vi "HT3_Open.vi"(8 "error in":errorcluster, 11 "File Path":path) -> (0 "error out":errorcluster, 1 "Num Records":i64, 2 "Header":T2={"Ident"="", "Format Version"="", "Creator Name"="", "Creator Version"="", "File Time"="", "Comment"="", "Binning"=0, "Offset"=0, "AcquisitionTime (ms)"=0, "HardwareSerial"=0, "SyncDivider"=0, "Resolution (ps)"=0.0, "InpRate0"=0, "InpRate1"=0, "CFD Settings"={"Sync Level"=150, "Sync ZeroX"=10, "Sync Offset"=-1000, "Chan Settings"=[{"CHx Level"=50, "CHx ZeroX"=10, "CHx Offset"=0}, {"CHx Level"=50, "CHx ZeroX"=10, "CHx Offset"=0}, {"CHx Level"=50, "CHx ZeroX"=10, "CHx Offset"=0}, {"CHx Level"=50, "CHx ZeroX"=10, "CHx Offset"=0}]}}, 3 "refnum out":refnum<file>, 4 "Stop After (ms)":i32, 5 "Stop Reason":enum16{"timeover", "manual", "overflow"}(ring), 7 "Image Header":T1)   [LabVIEW 2010]
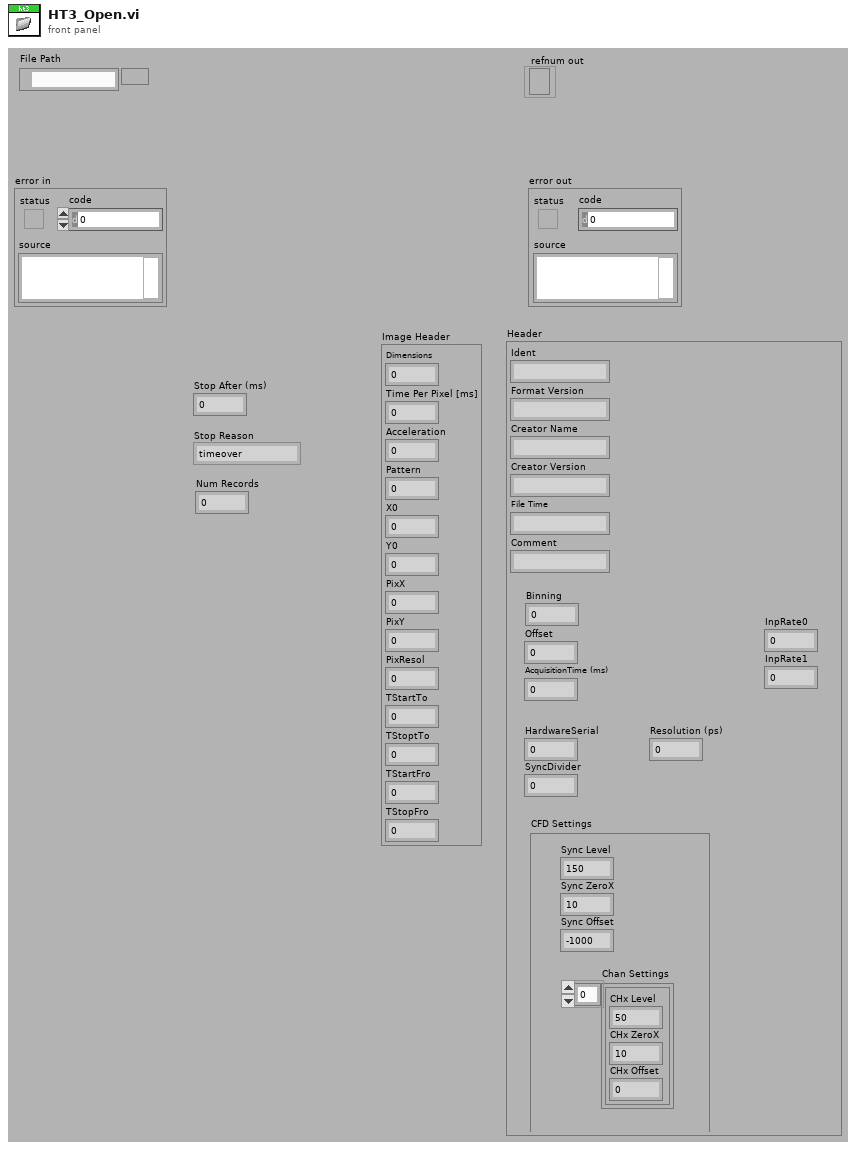
[diagram p1: front panel]
types:
  T1 = cluster{"Dimensions":i32, "Time Per Pixel [ms]":dbl, "Acceleration":i32, "Pattern":i32, "X0":sgl, "Y0":sgl, "PixX":i32, "PixY":i32, "PixResol":sgl, "TStartTo":sgl, "TStoptTo":sgl, "TStartFro":sgl, "TStopFro":sgl}
  T2 = cluster{"Ident":string, "Format Version":string, "Creator Name":string, "Creator Version":string, "File Time":string, "Comment":string, "Binning":i32, "Offset":i32, "AcquisitionTime (ms)":i32, "HardwareSerial":i32, "SyncDivider":i32, "Resolution (ps)":dbl, "InpRate0":i32, "InpRate1":i32, "CFD Settings":cluster{"Sync Level":i32, "Sync ZeroX":i32, "Sync Offset":i32, "Chan Settings":cluster{"CHx Level":i32, "CHx ZeroX":i32, "CHx Offset":i32}[]}}
  T3 = cluster{"Sync Level":i32, "Sync ZeroX":i32, "Sync Offset":i32, "Chan Settings":cluster{"CHx Level":i32, "CHx ZeroX":i32, "CHx Offset":i32}[]}
  T4 = enum16{"big-endian, network order", "native, host order", "little-endian"}
  T5 = enum16{"open", "replace", "create", "open or create", "replace or create", "replace or create with confirmation"}
  T6 = cluster{"Strings[0]":string, "Strings[1]":string, "Strings[2]":string, "Strings[3]":string, "Strings[4]":string, "Strings[5]":string}
  T7 = cluster{"[0]":i32, "[1]":i32, "[2]":i32, "[3]":i32}
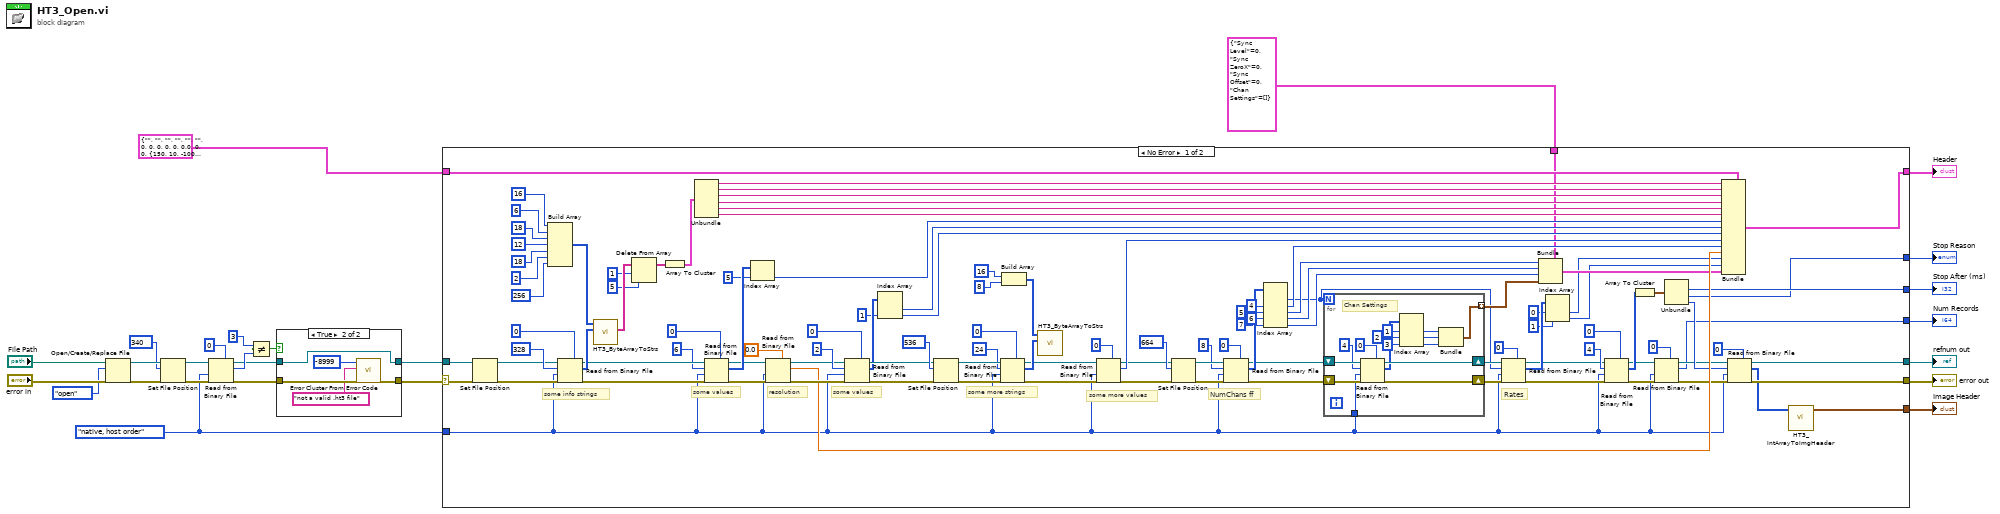
[diagram p0: block diagram]
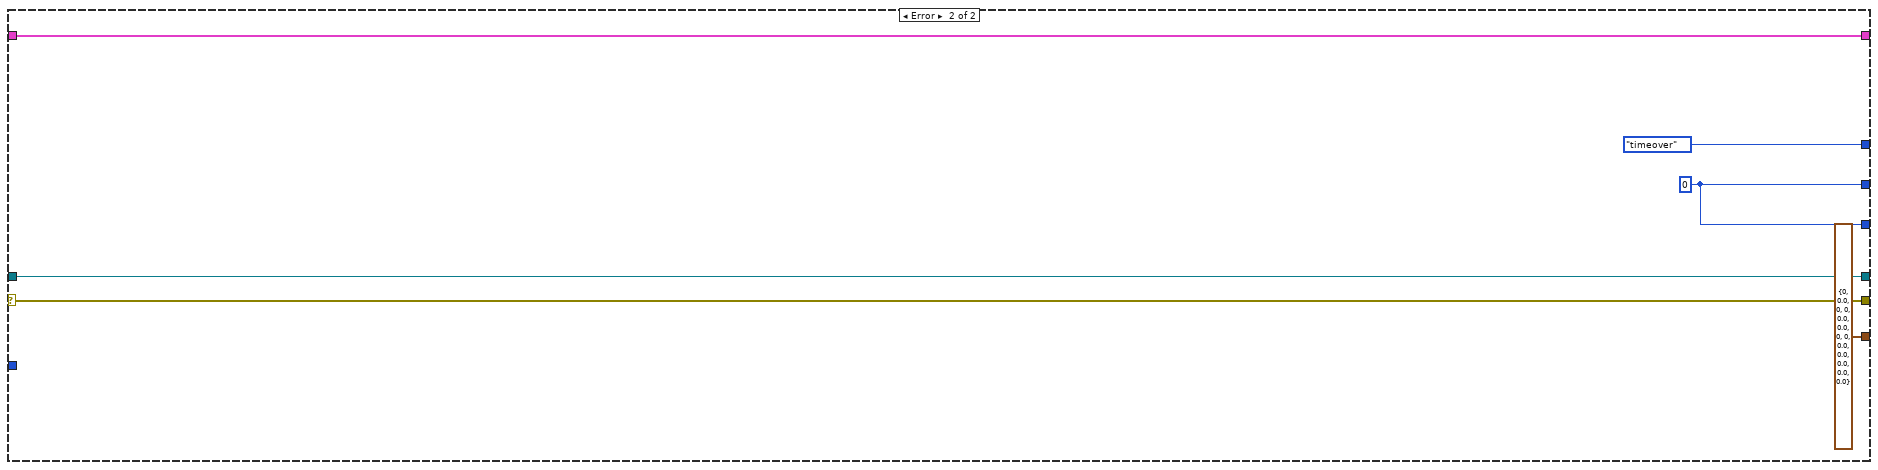
[diagram p3: hidden frame]
diagram:
  w12 = T4."native, host order" ("byte order (0:big-endian, network order)")
  n1 = Open/Create/Replace File(file path (use dialog)="File Path", error in="error in", operation (0:open)=T5."open") -> (refnum out=w15:refnum<file>, error out=w16:errorcluster)  [unwired: 4 out]
  n2 = Set File Position(offset (in bytes) (0)=i64 340, refnum=w15, error in=w16) -> (refnum out=w11:refnum<file>, error out=w13:errorcluster)  [unwired: 1 out]
  n3 = Read from Binary File(5:0, 8:w13, 9:w12, 11:w11) -> (0:w6:errorcluster, 2:w9:i32, 3:w3:refnum<file>)  [unwired: 3 out]
  n4 = Not Equal?(x=3, y=w9) -> (x != y?=w7:bool)
  n5 = case shown="True" w7 {
    tunnel: w6 -> [w28 w33]
    tunnel: [w28 w32] -> w5
    tunnel: [w27 w29] -> w4
    tunnel: w3 -> [w27 w29]
    frame False {
    }
    frame True {
      n6 = call <vilib>:"Error Cluster From Error Code.vi"("error in (no error)"=w33, "error message (\"\")"="not a valid .ht3 file" ("error message (\"\")"), "error code (0)"=-8999) -> ("error out"=w32:errorcluster)  [unwired: 1 in, 5 out]
    }
  }
  n7 = case shown="No Error" w5 {
    selector: w5 -> [w129 w167]
    tunnel: [w94 w167] -> w23
    tunnel: [w93 w166] -> w22
    tunnel: w4 -> [w127 w166]
    tunnel: w12 -> [w38 _]
    tunnel: [w120 w163] -> w21
    tunnel: [w41 enum16{"timeover", "manual", "overflow"}."timeover" ("Stop Reason")] -> w20
    tunnel: [w42 w164] -> w19
    tunnel: [w34 w164] -> w18
    tunnel: T2 {"Ident"="", "Format Version"="", "Creator Name"="", "Creator Version"="", "File Time"="", "Comment"="", "Binning"=0, "Offset"=0, "AcquisitionTime (ms)"=0, "HardwareSerial"=0, "SyncDivider"=0, "Resolution (ps)"=0.0, "InpRate0"=0, "InpRate1"=0, "CFD Settings"={"Sync Level"=150, "Sync ZeroX"=10, "Sync Offset"=-1000, "Chan Settings"=[{"CHx Level"=50, "CHx ZeroX"=10, "CHx Offset"=0}, {"CHx Level"=50, "CHx ZeroX"=10, "CHx Offset"=0}, {"CHx Level"=50, "CHx ZeroX"=10, "CHx Offset"=0}, {"CHx Level"=50, "CHx ZeroX"=10, "CHx Offset"=0}]}} ("Header") -> [w121 w163]
    tunnel: [w91 T1 {"Dimensions"=0, "Time Per Pixel [ms]"=0.0, "Acceleration"=0, "Pattern"=0, "X0"=0.0, "Y0"=0.0, "PixX"=0, "PixY"=0, "PixResol"=0.0, "TStartTo"=0.0, "TStoptTo"=0.0, "TStartFro"=0.0, "TStopFro"=0.0} ("Image Header")] -> w2
    tunnel: T3 {"Sync Level"=0, "Sync ZeroX"=0, "Sync Offset"=0, "Chan Settings"=[]} ("CFD Settings") -> [w63 _]
    frame No Error {
      # "Rates"
      # "NumChans ff"
      # "some values"
      # "resolution"
      # "some more values"
      # "some more strings"
      # "some values"
      # "some info strings"
      n8 = Set File Position(refnum=w127, error in=w129) -> (refnum out=w126:refnum<file>, error out=w128:errorcluster)  [unwired: 2 out]
      n9 = Build Array(16 ("Length"), 6 ("Length"), 18 ("Length"), 12 ("Length"), 18 ("Length"), 2 ("Length"), 256 ("Length")) -> (w136:i32[])
      n10 = Read from Binary File(5:u8 0, 8:w128, 9:w38, 10:328 ("count (1)"), 11:w126) -> (0:w131:errorcluster, 2:w144:u8[], 3:w130:refnum<file>)  [unwired: 2 out]
      n11 = call "HT3_ByteArrayToStrs.vi"("Byte Array"=w144, "Lengths"=w136) -> ("Strings"=w135:string[])  [unwired: 9 out]
      n12 = Delete From Array(array=w135, length=1, index=5) -> (array with subset deleted=w132:string[])  [unwired: 1 out]
      n13 = Array To Cluster(array=w132) -> (cluster=w119:T6)
      n14 = Unbundle(w119) -> ("Strings[0]"=w118:string, "Strings[1]"=w117:string, "Strings[2]"=w116:string, "Strings[3]"=w115:string, "Strings[4]"=w114:string, "Strings[5]"=w113:string)
      n15 = Read from Binary File(5:0, 8:w131, 9:w38, 10:6 ("count (1)"), 11:w130) -> (0:w89:errorcluster, 2:w123:i32[], 3:w88:refnum<file>)  [unwired: 2 out]
      n16 = Index Array(array=w123, index=5) -> (element=w112:i32)
      n17 = Read from Binary File(5:0.0 ("Resolution (ns)"), 8:w89, 9:w38, 11:w88) -> (0:w85:errorcluster, 2:w77:dbl, 3:w83:refnum<file>)  [unwired: 1 in, 2 out]
      n18 = Read from Binary File(5:0, 8:w85, 9:w38, 10:2 ("count (1)"), 11:w83) -> (0:w84:errorcluster, 2:w81:i32[], 3:w82:refnum<file>)  [unwired: 1 in, 1 out]
      n19 = Index Array(array=w81, index #2=1 ("index")) -> (element #1=w79:i32, element #2=w78:i32)  [unwired: 1 in]
      n20 = Set File Position(offset (in bytes) (0)=i64 536, refnum=w82, error in=w84) -> (refnum out=w109:refnum<file>, error out=w110:errorcluster)  [unwired: 1 out]
      n21 = Read from Binary File(5:u8 0, 8:w110, 9:w38, 10:24 ("count (1)"), 11:w109) -> (0:w102:errorcluster, 2:w106:u8[], 3:w101:refnum<file>)  [unwired: 2 out]
      n22 = Build Array(16 ("Length"), 8 ("Length")) -> (w103:i32[])
      n23 = call "HT3_ByteArrayToStrs.vi"("Byte Array"=w106, "Lengths"=w103) -> ()  [unwired: 10 out]
      n24 = Read from Binary File(5:0, 8:w102, 9:w38, 11:w101) -> (0:w74:errorcluster, 2:w76:i32, 3:w73:refnum<file>)  [unwired: 1 in, 2 out]
      n25 = Set File Position(offset (in bytes) (0)=i64 664, refnum=w73, error in=w74) -> (refnum out=w70:refnum<file>, error out=w71:errorcluster)  [unwired: 1 out]
      n26 = Read from Binary File(5:0, 8:w71, 9:w38, 10:8 ("count (1)"), 11:w70) -> (0:w67:errorcluster, 2:w68:i32[], 3:w64:refnum<file>)  [unwired: 2 out]
      n27 = Index Array(array=w68, index #2=4 ("index"), index #3=5 ("index"), index #4=6 ("index"), index #5=7 ("index")) -> (element #1=w50:i32, element #2=w65:i32, element #3=w58:i32, element #4=w57:i32, element #5=w59:i32)  [unwired: 1 in]
      n28 = for {
        N: w50 -> [_]
        shift-right: [w160] -> w54
        shift-left: w67 -> [w161]
        tunnel: w38 -> [w159]
        shift-right: [w157] -> w52
        shift-left: w64 -> [w158]
        tunnel: [w147] -> w56 mode=indexing
        # "Chan Settings"
        n29 = Read from Binary File(5:0, 8:w161, 9:w159, 10:4 ("count (1)"), 11:w158) -> (0:w160:errorcluster, 2:w154:i32[], 3:w157:refnum<file>)  [unwired: 1 in, 1 out]
        n30 = Index Array(array=w154, index #1=1 ("index"), index #2=2 ("index"), index #3=3 ("index")) -> (element #1=w150:i32, element #2=w149:i32, element #3=w148:i32)
        n31 = Bundle(w150, w149, w148) -> (w147:cluster{i32, i32, i32})  [unwired: 1 in]
      }
      n32 = Read from Binary File(5:0, 8:w54, 9:w38, 10:w50, 11:w52) -> (0:w53:errorcluster, 2:w49:i32[], 3:w44:refnum<file>)  [unwired: 2 out]
      n33 = Bundle(cluster=w63, "Sync Level"=w58, "Sync ZeroX"=w57, "Sync Offset"=w59, "Chan Settings"=w56) -> (w55:T3)
      n34 = Index Array(array=w49, index #1=0 ("index"), index #2=1 ("index")) -> (element #1=w46:i32, element #2=w45:i32)
      n35 = Read from Binary File(5:0, 8:w53, 9:w38, 10:4 ("count (1)"), 11:w44) -> (0:w40:errorcluster, 2:w96:i32[], 3:w37:refnum<file>)  [unwired: 2 out]
      n36 = Array To Cluster(array=w96) -> (cluster=w97:T7)
      n37 = Read from Binary File(5:i64 0, 8:w40, 9:w38, 11:w37) -> (0:w39:errorcluster, 2:w34:i64, 3:w36:refnum<file>)  [unwired: 1 in, 2 out]
      n38 = Unbundle(w97) -> ("[1]"=w42:i32, "[2]"=w41:i32, "[3]"=w43:i32)  [unwired: 1 out]
      n39 = Bundle(cluster=w121, "Ident"=w118, "Format Version"=w117, "Creator Name"=w116, "Creator Version"=w115, "File Time"=w114, "Comment"=w113, "Binning"=w112, "Offset"=w79, "AcquisitionTime (ms)"=w78, "HardwareSerial"=w76, "SyncDivider"=w65, "Resolution (ps)"=w77, "InpRate0"=w46, "InpRate1"=w45, "CFD Settings"=w55) -> (w120:T2)
      n40 = Read from Binary File(5:0, 8:w39, 9:w38, 10:w43, 11:w36) -> (0:w94:errorcluster, 2:w92:i32[], 3:w93:refnum<file>)  [unwired: 2 out]
      n41 = call "HT3_IntArrayToImgHeader.vi"("Array"=w92) -> ("Image Header"=w91:T1)  [unwired: 10 out]
    }
    frame Error {
      w164 = 0 ("Stop After (ms)")
    }
  }
  "refnum out" <- w22
  "error out" <- w23
  "Header" <- w21
  "Stop Reason" <- w20
  "Stop After (ms)" <- w19
  "Num Records" <- w18
  "Image Header" <- w2
